vi "Flock_LoggerException.vi"(8 "Error In":errorcluster, 11 "Process List":T1) -> (0 "Error Out":errorcluster)   [LabVIEW 2014, in "Logger.lvlib"]
uses:
  Logger.lvlib
  Shared Code/AMC/VI Source/CentralProcessMessaging/Flock_Shared_CentralProcessMessaging.lvlib
  Shared Code/AMC/VI Source/Error Handling/Flock_ErrorHandling.lvlib
  Shared Code/AMC/VI Source/LocalProcessMessaging/Flock_Shared_LocalProcessMessaging.lvlib
  Shared Code/AMC/VI Source/ProcessList.ctl
  Shared Code/AMC/VI Source/Flock_Shared_Messaging.lvlib
panel:
  out "resulting string":string
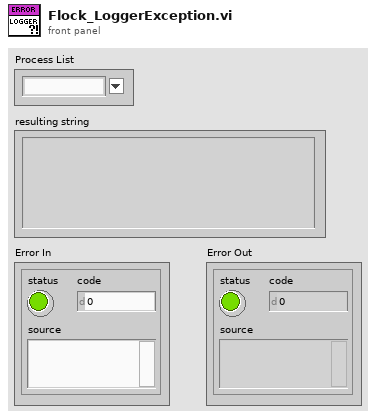
[diagram p1: front panel]
types:
  T1 = typedef "Flock_Shared_Messaging.lvlib/ProcessList.ctl" = string
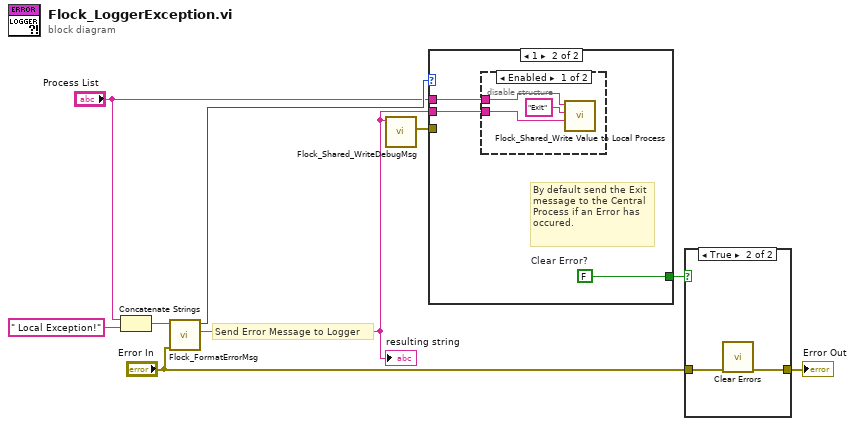
[diagram p0: block diagram]
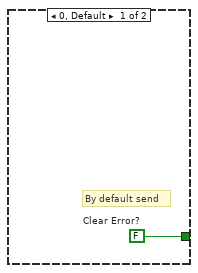
[diagram p3: hidden frame]
diagram:
  # "Send Error Message to Logger"
  n1 = Concatenate Strings("Process List", " Local Exception!" ("initial string")) -> (w1:string)
  n2 = call "Flock_FormatErrorMsg.vi"("error in (no error)"="Error In", "initial string"=w1) -> ("String"=w9:string, "code"=w8:i32)  [unwired: 8 in]
  "resulting string" <- w9
  n3 = call "Flock_Shared_WriteDebugMsg.vi"("Current Message Case"=w9) -> ("error out"=w4:errorcluster)  [unwired: 10 in]
  n4 = case shown="1" w8 {
    tunnel: w9 -> [_ w11]
    tunnel: [w10 w13] -> w7
    tunnel: w4 -> [_ _]
    tunnel: "Process List" -> [_ w12]
    frame 0, Default {
      w10 = FALSE  # Clear Error?
      # "By default send"
    }
    frame 1 {
      w13 = FALSE  # Clear Error?
      # "By default send the Exit message to the Central Process if an Error has occured."
      n5 = disable-structure shown="Enabled" {
        disable-tunnel: w12 -> [w16 _]
        disable-tunnel: w11 -> [w14 _]
        frame Enabled {
          n6 = call "Flock_Shared_Write Value to Local Process.vi"("Message Value"=w14, "Message Name"="Exit", "Process List"=w16) -> ()  [unwired: 8 in, 1 out]
        }
        frame Disabled {
        }
      }
    }
  }
  n7 = case shown="True" w7 {
    tunnel: "Error In" -> [w17 w19]
    tunnel: [w17 w18] -> w5
    frame False {
    }
    frame True {
      n8 = call <vilib>:"Clear Errors.vi"("error in (no error)"=w19) -> ("error out"=w18:errorcluster)  [unwired: 5 in, 1 out]
    }
  }
  "Error Out" <- w5
